vi "Get Computer Metadata.vi"(8 "error in (no error)":errorcluster) -> (0 "error out":errorcluster, 3 "Computer Metadata":T1)   [LabVIEW 2023]
doc: "This VI opens a reference to the localhost resource, gets computer OS and hardware metadata, then builds the \"Computer Metadata\" cluster from it."
uses:
  Type Definitions/Computer Metadata.ctl
  Type Definitions/Payload Class.ctl
  Type Definitions/Enum - Metadata.ctl
  <vilib>/Utility/error.llb/Trim Whitespace One-Sided.vi
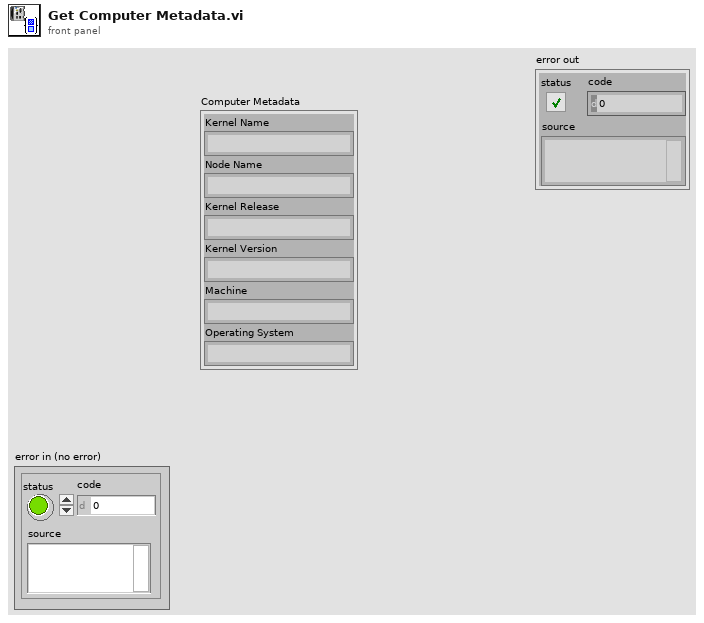
[diagram p1: front panel]
types:
  T1 = typedef "Computer Metadata.ctl" = cluster{"Kernel Name":string, "Node Name":string, "Kernel Release":string, "Kernel Version":string, "Machine":string, "Operating System":string}
  T2 = typedef "Enum - Metadata.ctl" = enum16{"Computer Metadata", "Computer Resources", "RT Image Metadata", "Startup Settings", "Telemetry Recorder Status"}
  T3 = typedef "Payload Class.ctl" = enum16{"System State", "Parameters", "Metadata", "Software Monitor", "Data", "Commands"}
  T4 = cluster{"[0]":string, "[1]":string, "[2]":string, "[3]":string, "[4]":string, "[5]":string}
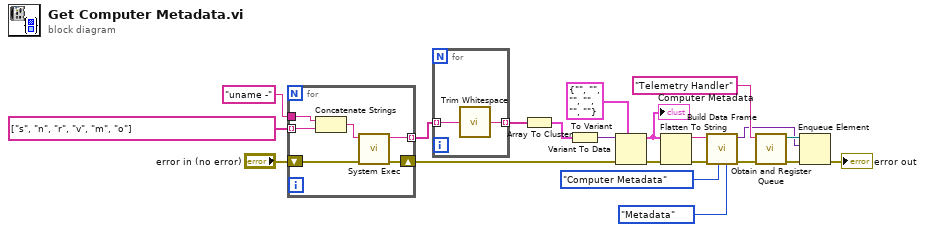
[diagram p0: block diagram]
diagram:
  n1 = for {
    tunnel: "uname -" ("command line") -> [w27]
    tunnel: [w25] -> w2 mode=indexing
    tunnel: string[] ["s", "n", "r", "v", "m", "o"] ("string") -> [w24] mode=indexing
    shift-right: [w22] -> w12
    shift-left: "error in (no error)" -> [w23]
    n2 = Concatenate Strings(w27, w24) -> (w26:string)
    n3 = call <vilib>:"System Exec.vi"("error in (no error)"=w23, "command line"=w26) -> ("error out"=w22:errorcluster, "standard output"=w25:string)  [unwired: 6 in, 2 out]
  }
  n4 = for {
    tunnel: w2 -> [w29] mode=indexing
    tunnel: [w28] -> w1 mode=indexing
    n5 = call <vilib>:"Trim Whitespace.vi"("string"=w29) -> ("trimmed string"=w28:string)  [unwired: 1 in]
  }
  n6 = Array To Cluster(array=w1) -> (cluster=w18:T4)
  n7 = To Variant(anything=w18) -> (Variant=w17:variant)
  n8 = Variant To Data(error in=w12, type=T1 {"Kernel Name"="", "Node Name"="", "Kernel Release"="", "Kernel Version"="", "Machine"="", "Operating System"=""} ("Computer Metadata"), Variant=w17) -> (data=w10:T1, error out=w11:errorcluster)
  "Computer Metadata" <- w10
  n9 = Flatten To String(anything=w10, error in (no error)=w11) -> (data string=w15:string, error out=w6:errorcluster)  [unwired: 2 in, 1 out]
  n10 = call "Build Data Frame.vi"("Payload Class (Data)"=Payload_Class."Metadata", "Payload ID (0)"=Enum_-_Metadata."Computer Metadata" ("Metadata"), "error in (no error)"=w6, "Payload (Empty String)"=w15) -> ("error out"=w5:errorcluster, "Frame"=w4:variant)  [unwired: 6 in]
  n11 = call "Obtain and Register Queue.vi"("error in (no error)"=w5, "Queue Name (unnamed)"="Telemetry Handler" ("name (unnamed)")) -> ("error out"=w9:errorcluster, "Queue Reference"=w8:refnum<queue>)  [unwired: 8 in]
  n12 = Enqueue Element(queue=w8, element=w4, error in (no error)=w9) -> (error out=→"error out":errorcluster)  [unwired: 1 in, 2 out]
